vi "Test 2.vi"   [LabVIEW 2020, in "allgemeine Sub-VIs.lvlib"]
uses:
  allgemeine Sub-VIs.lvlib
  AK-Schnittstelle/Aktionen AK.ctl
  AK-Schnittstelle/Aktionen Gespeicherte Werte.ctl
  Zykluszeiterfassung Aktionen.ctl
  AK-Schnittstelle/AK-Schnittstelle.lvlib
  AK-Schnittstelle/AK TCP/AK TCP.lvlib
types:
  T1 = typedef "AK-Schnittstelle.lvlib/Aktionen AK.ctl" = enum16{"lesen", "initialisieren", "beenden", "AK Komm"}
  T2 = typedef "allgemeine Sub-VIs.lvlib/Zykluszeiterfassung Aktionen.ctl" = enum16{"lesen", "init", "Messdaten1", "ToolWeb", "AK FT-IR", "AK Extern", "AK Amium"}
  T3 = typedef "AK-Schnittstelle.lvlib/Aktionen Gespeicherte Werte.ctl" = enum16{"lesen", "laden", "speichern", "Seriell", "TCP", "Diverse", "AKTIV", "AK-Namen"}
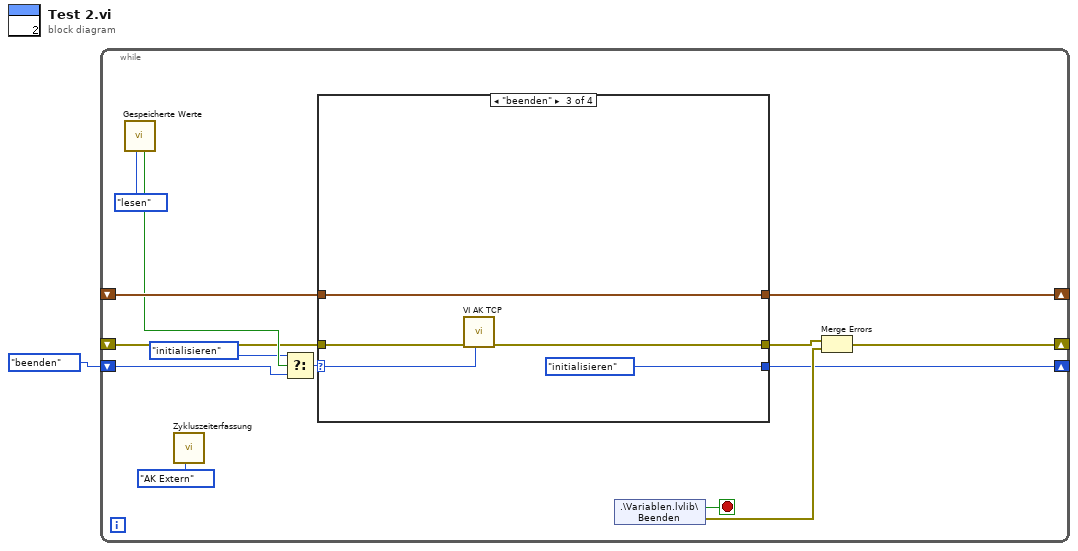
[diagram p0: block diagram]
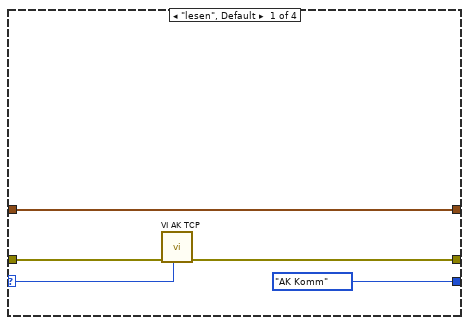
[diagram p2: hidden frame]
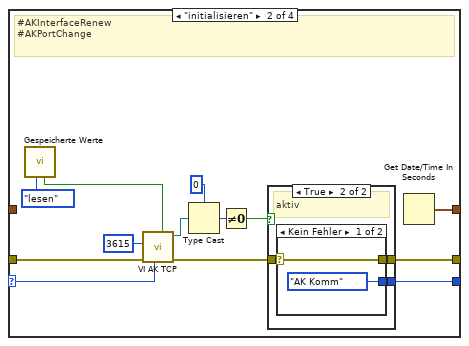
[diagram p3: hidden frame]
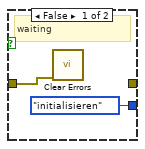
[diagram p4: hidden frame]
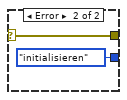
[diagram p5: hidden frame]
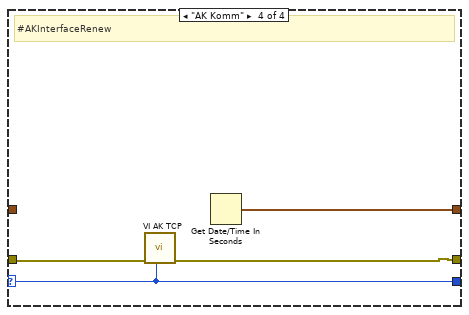
[diagram p6: hidden frame]
diagram:
  n1 = while {
    shift-right: [w4] -> _
    shift-left: Aktionen_AK."beenden" ("Aktionen") -> [w15]
    shift-right: [w14] -> _
    shift-left: _ -> [w13]
    shift-right: [w6] -> _
    shift-left: _ -> [w5]
    stop <- w11 stop-if-true
    n2 = call "Gespeicherte Werte.vi"("Aktionen"=Aktionen_Gespeicherte_Werte."lesen") -> ("Port changed out"=w9:bool)  [unwired: 6 in, 4 out]
    n3 = call "Zykluszeiterfassung.vi"("Aktionen"=Zykluszeiterfassung_Aktionen."AK Extern") -> ()  [unwired: 10 in, 1 out]
    n4 = Select(t=Aktionen_AK."initialisieren" ("Aktionen"), s=w9, f=w15) -> (s? t:f=w2:T1)
    n5 = case shown="\"beenden\"" w2 {
      selector: w2 -> [w18 w32 w46 w50]
      tunnel: [Aktionen_AK."AK Komm" ("Aktionen") w30 Aktionen_AK."initialisieren" ("Aktionen") w50] -> w4
      tunnel: [w19 w29 w45 w51] -> w14
      tunnel: w13 -> [w19 _ w45 _]
      tunnel: [w16 w25 w43 w48] -> w3
      tunnel: w5 -> [w17 w24 w44 w49]
      frame "lesen", Default {
        n6 = call "VI AK TCP.vi"("Aktionen"=w18, "error in"=w17) -> ("error out"=w16:errorcluster)  [unwired: 8 in, 1 out]
      }
      frame "initialisieren" {
        # "#AKInterfaceRenew\n#AKPortChange"
        n7 = call "Gespeicherte Werte.vi"("Aktionen"=Aktionen_Gespeicherte_Werte."lesen") -> ("Port changed out"=w22:bool)  [unwired: 6 in, 4 out]
        n8 = call "VI AK TCP.vi"("Port changed in"=w22, "Aktionen"=w32, "error in"=w24, "Port"=u16 3615) -> ("error out"=w31:errorcluster, "connection ID"=w23:refnum<k5>)  [unwired: 6 in]
        n9 = Type Cast(type=u32 0, x=w23) -> (*(type *) &x=w27:u32)
        n10 = Not Equal To 0?(x=w27) -> (x != 0?=w26:bool)
        n11 = case shown="True" w26 {
          tunnel: w31 -> [w35 w38]
          tunnel: [Aktionen_AK."initialisieren" ("Aktionen") w37] -> w30
          tunnel: [_ w36] -> w25
          frame False {
            # "waiting"
            n12 = call <vilib>:"Clear Errors.vi"("error in (no error)"=w35) -> ()  [unwired: 5 in, 2 out]
          }
          frame True {
            # "aktiv"
            n13 = case shown="Kein Fehler" w38 {
              selector: w38 -> [w39 w41]
              tunnel: [Aktionen_AK."AK Komm" ("Aktionen") Aktionen_AK."initialisieren" ("Aktionen")] -> w37
              tunnel: [w39 w41] -> w36
              frame No Error {
              }
              frame Error {
              }
            }
          }
        }
        n14 = Get Date/Time In Seconds() -> (seconds since 1Jan1904=w29:timestamp)
      }
      frame "beenden" {
        n15 = call "VI AK TCP.vi"("Aktionen"=w46, "error in"=w44) -> ("error out"=w43:errorcluster)  [unwired: 8 in, 1 out]
      }
      frame "AK Komm" {
        # "#AKInterfaceRenew"
        n16 = call "VI AK TCP.vi"("Aktionen"=w50, "error in"=w49) -> ("error out"=w48:errorcluster)  [unwired: 8 in, 1 out]
        n17 = Get Date/Time In Seconds() -> (seconds since 1Jan1904=w51:timestamp)
      }
    }
    n18 = shared-variable ".\\Variablen.lvlib\\Beenden"() -> (w11:bool, error out=w7:errorcluster)  [unwired: 1 in]
    n19 = Merge Errors(w3, w7) -> (w6:errorcluster)
  }
